vi "User.File.Read.vi"(8 "error in (no error)":errorcluster) -> (0 "error out":errorcluster)   [LabVIEW 2013]
uses:
  User.Level.ctl
  User.Info.ctl
  User.Global.vi
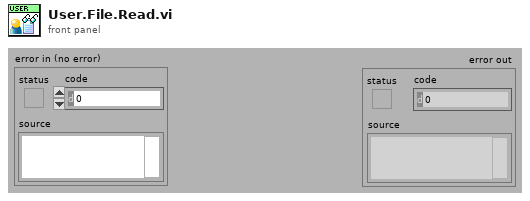
[diagram p1: front panel]
types:
  T1 = typedef "User.Info.ctl" = cluster{"ID":i32, "Name":string, "Pass":string, "Level":T2, "Del":bool}
  T2 = typedef "User.Level.ctl" = enum16{"-", "Operator", "Technician", "Administrator"}
  T3 = cluster{"Users":T1[], "Temp":string, "TS":timestamp, "Operator":string, "User":string, "Duration":dbl}
  T4 = cluster{"f":u8[], "u":u8[], "c":u8[][], "k":u8[][], "u2":u8[][]}
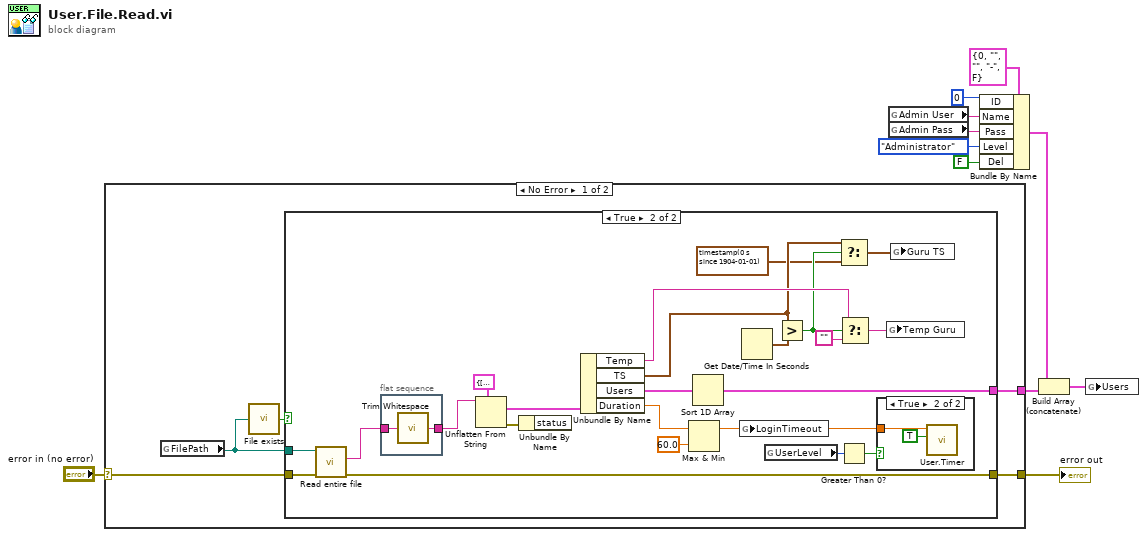
[diagram p0: block diagram]
diagram:
  n1 = case shown="No Error" "error in (no error)" {
    selector: "error in (no error)" -> [w15 w175]
    tunnel: [w16 w175] -> w10
    tunnel: [w13 _] -> w2
    frame No Error {
      n2 = global read "User.Global.vi" "FilePath"() -> (w12:path)
      n3 = call "File exists.vi"("file path"=w12) -> ("exists?"=w14:bool)  [unwired: 4 in]
      n4 = case shown="True" w14 {
        tunnel: [w17 w40] -> w16
        tunnel: w15 -> [w17 w39]
        tunnel: w12 -> [_ w38]
        tunnel: [_ w23] -> w13
        frame False {
        }
        frame True {
          n5 = call "Read entire file.vi"("error in"=w39, "file"=w38) -> ("error out"=w40:errorcluster, "contents"=w24:string)  [unwired: 4 in]
          n6 = flat-sequence {
            tunnel: w24 -> [w44]
            tunnel: [w43] -> w37
            frame #0 {
              n7 = disable-structure shown="Enabled" {
                disable-tunnel: [w46 w174] -> w43
                disable-tunnel: w44 -> [w45 w174]
                frame Enabled {
                  w52 = 16 ("length (rest)")
                  n8 = Unbundle By Name(T4 {"f"=[99, 124, 119, 123, 242, 107, 111, 197, 48, 1, 103, 43, 254, 215, 171, 118, 202, 130, 201, 125, 250, 89, 71, 240, 173, 212, 162, 175, 156, 164, 114, 192, 183, 253, 147, 38, 54, 63, 247, 204, 52, 165, 229, 241, 113, 216, 49, 21, 4, 199, 35, 195, 24, 150, 5, 154, 7, 18, 128, 226, 235, 39, 178, 117, 9, 131, 44, 26, 27, 110, 90, 160, 82, 59, 214, 179, 41, 227, 47, 132, 83, 209, 0, 237, 32, 252, 177, 91, 106, 203, 190, 57, 74, 76, 88, 207, 208, 239, 170, 251, 67, 77, 51, 133, 69, 249, 2, 127, 80, 60, 159, 168, 81, 163, 64, 143, 146, 157, 56, 245, 188, 182, 218, 33, 16, 255, 243, 210, 205, 12, 19, 236, 95, 151, 68, 23, 196, 167, 126, 61, 100, 93, 25, 115, 96, 129, 79, 220, 34, 42, 144, 136, 70, 238, 184, 20, 222, 94, 11, 219, 224, 50, 58, 10, 73, 6, 36, 92, 194, 211, 172, 98, 145, 149, 228, 121, 231, 200, 55, 109, 141, 213, 78, 169, 108, 86, 244, 234, 101, 122, 174, 8, 186, 120, 37, 46, 28, 166, 180, 198, 232, 221, 116, 31, 75, 189, 139, 138, 112, 62, 181, 102, 72, 3, 246, 14, 97, 53, 87, 185, 134, 193, 29, 158, 225, 248, 152, 17, 105, 217, 142, 148, 155, 30, 135, 233, 206, 85, 40, 223, 140, 161, 137, 13, 191, 230, 66, 104, 65, 153, 45, 15, 176, 84, 187, 22], "u"=[82, 9, 106, 213, 48, 54, 165, 56, 191, 64, 163, 158, 129, 243, 215, 251, 124, 227, 57, 130, 155, 47, 255, 135, 52, 142, 67, 68, 196, 222, 233, 203, 84, 123, 148, 50, 166, 194, 35, 61, 238, 76, 149, 11, 66, 250, 195, 78, 8, 46, 161, 102, 40, 217, 36, 178, 118, 91, 162, 73, 109, 139, 209, 37, 114, 248, 246, 100, 134, 104, 152, 22, 212, 164, 92, 204, 93, 101, 182, 146, 108, 112, 72, 80, 253, 237, 185, 218, 94, 21, 70, 87, 167, 141, 157, 132, 144, 216, 171, 0, 140, 188, 211, 10, 247, 228, 88, 5, 184, 179, 69, 6, 208, 44, 30, 143, 202, 63, 15, 2, 193, 175, 189, 3, 1, 19, 138, 107, 58, 145, 17, 65, 79, 103, 220, 234, 151, 242, 207, 206, 240, 180, 230, 115, 150, 172, 116, 34, 231, 173, 53, 133, 226, 249, 55, 232, 28, 117, 223, 110, 71, 241, 26, 113, 29, 41, 197, 137, 111, 183, 98, 14, 170, 24, 190, 27, 252, 86, 62, 75, 198, 210, 121, 32, 154, 219, 192, 254, 120, 205, 90, 244, 31, 221, 168, 51, 136, 7, 199, 49, 177, 18, 16, 89, 39, 128, 236, 95, 96, 81, 127, 169, 25, 181, 74, 13, 45, 229, 122, 159, 147, 201, 156, 239, 160, 224, 59, 77, 174, 42, 245, 176, 200, 235, 187, 60, 131, 83, 153, 97, 23, 43, 4, 126, 186, 119, 214, 38, 225, 105, 20, 99, 85, 33, 12, 125], "c"=[[90, 1, 69, 10], [61, 7, 207, 135], [244, 76, 178, 236], [74, 228, 164, 36], [49, 56, 198, 20], [216, 46, 208, 179], [133, 132, 236, 77], [207, 242, 209, 46], [50, 72, 115, 220], [12, 63, 9, 147], [44, 98, 98, 95], [207, 96, 72, 105], [186, 6, 247, 158], [234, 102, 163, 111], [137, 187, 229, 222], [227, 144, 179, 113], [230, 26, 138, 86], [182, 57, 254, 13], [198, 4, 193, 48], [70, 219, 173, 183], [210, 107, 84, 143], [12, 124, 41, 57], [63, 130, 27, 211], [37, 148, 114, 65], [79, 143, 35, 12], [100, 82, 170, 130], [202, 120, 232, 9], [121, 89, 182, 100], [208, 43, 215, 176], [67, 243, 10, 53], [91, 208, 177, 81], [239, 236, 154, 72], [196, 193, 96, 186], [180, 121, 125, 50], [137, 139, 226, 60], [34, 137, 7, 53], [158, 147, 133, 111], [135, 50, 106, 143], [239, 169, 204, 99], [102, 103, 120, 116], [120, 4, 246, 41], [42, 234, 248, 93], [14, 185, 136, 179], [205, 32, 203, 86], [45, 47, 23, 92], [255, 54, 156, 166], [197, 67, 52, 62], [104, 222, 240, 199], [163, 27, 71, 148], [7, 197, 239, 1], [241, 143, 20, 21], [8, 99, 255, 104], [232, 163, 209, 25], [92, 45, 219, 50], [194, 134, 219, 63], [153, 81, 228, 210], [243, 13, 2, 164], [239, 102, 62, 24], [173, 162, 207, 39], [202, 229, 36, 87], [116, 202, 100, 247], [175, 32, 217, 150], [45, 224, 229, 39], [52, 243, 43, 245]], "k"=[[2, 3, 1, 1], [1, 2, 3, 1], [1, 1, 2, 3], [3, 1, 1, 2]], "u2"=[[14, 11, 13, 9], [9, 14, 11, 13], [13, 9, 14, 11], [11, 13, 9, 14]]} ("Cipher Keys")) -> ("c"=w56:u8[][], "u"=w58:u8[], "u2"=w55:u8[][])
                  n9 = String To Byte Array(string=w45) -> (unsigned byte array=w50:u8[])
                  n10 = Array Size(array=w50) -> (size(s)=w49:i32)
                  n11 = Divide(x=w49, y=w52) -> (x/y=w51:dbl)
                  n12 = Round Toward +Infinity(x=w51) -> (ceil(x): smallest int >= x=w53:dbl)
                  n13 = Reshape Array(w50, w53, w52) -> (w54:u8[][])
                  n14 = for {
                    tunnel: w54 -> [w63] mode=indexing
                    tunnel: w55 -> [w88]
                    tunnel: w56 -> [w66]
                    tunnel: [w83] -> w57 mode=indexing
                    tunnel: w58 -> [w82]
                    shift-right: [w64] -> _
                    shift-left: u8[] [0, 0, 0, 0, 0, 0, 0, 0, 0, 0, 0, 0, 0, 0, 0, 0] ("initialized array") -> [w62]
                    tunnel: TRUE ("Cipher Block Chaining (CBC)") -> [w61]
                    w91 = 4 ("index")
                    n15 = Array Size(array=w66) -> (size(s)=w68:i32[])
                    n16 = Index Array(array=w68, index=0) -> (element=w70:i32)
                    n17 = expression code="x-4"(w70) -> (w67:i32)
                    n18 = Reshape Array(w63, w91, w91) -> (w80:u8[][])
                    n19 = Array Subset(array=w66, index (row)=w67, length (col)=4 ("length")) -> (w79:u8[][])  [unwired: 2 in]
                    n20 = Transpose 2D Array(2D array=w79) -> (transposed array=w77:u8[][])
                    n21 = Exclusive Or ("add_round_key")(1:w77, 2:w80) -> (0:w78:u8[][])
                    n22 = for {
                      N: 9 -> [_]
                      tunnel: w88 -> [w108]
                      shift-right: [w106] -> w76
                      shift-left: w78 -> [w112]
                      tunnel: w66 -> [w114]
                      tunnel: [w114] -> w85
                      tunnel: [w113] -> w81
                      tunnel: w82 -> [w113]
                      i -> [w117]
                      n23 = for "inv_shift_rows" {
                        tunnel: w112 -> [w167] mode=indexing
                        tunnel: [w166] -> w111 mode=indexing
                        i -> [w165]
                        n24 = Rotate 1D Array(1:w167, 2:w165) -> (0:w166:u8[])
                      }
                      n25 = for "inv_sub_bytes" {
                        tunnel: w113 -> [w170]
                        tunnel: w111 -> [w169] mode=indexing
                        tunnel: [w168] -> w110 mode=indexing
                        n26 = for {
                          tunnel: w170 -> [w173]
                          tunnel: w169 -> [w172] mode=indexing
                          tunnel: [w171] -> w168 mode=indexing
                          n27 = Index Array(array=w173, index=w172) -> (element=w171:u8)
                        }
                      }
                      n28 = expression code="4*(9-x)"(w117) -> (w116:i32)
                      n29 = Array Subset(array=w114, index (row)=w116, length (col)=4 ("length")) -> (w119:u8[][])  [unwired: 2 in]
                      n30 = Transpose 2D Array(2D array=w119) -> (transposed array=w115:u8[][])
                      n31 = Exclusive Or(1:w115, 2:w110) -> (0:w107:u8[][])
                      n32 = Transpose 2D Array(2D array=w107) -> (transposed array=w109:u8[][])
                      n33 = for "mix_columns" {
                        tunnel: w108 -> [w122] mode=indexing
                        tunnel: w109 -> [w120]
                        tunnel: [w121] -> w106 mode=indexing
                        n34 = for {
                          tunnel: w122 -> [w126]
                          tunnel: [w124] -> w121 mode=indexing
                          tunnel: w120 -> [w123] mode=indexing
                          n35 = for {
                            tunnel: w126 -> [w130] mode=indexing
                            shift-right: [w139] -> w124
                            shift-left: u8 0 -> [w128]
                            tunnel: w123 -> [w131] mode=indexing
                            n36 = To Unsigned Word Integer(number=w131) -> (unsigned 16bit integer=w132:u16)
                            n37 = Number To Boolean Array(number=w130) -> (Boolean array=w133:bool[])
                            n38 = for {
                              N: 8 -> [_]
                              shift-right: [w157] -> w134
                              shift-left: u16 0 ("prod") -> [w158]
                              tunnel: w133 -> [w155] mode=indexing
                              tunnel: w132 -> [w154]
                              i -> [w156]
                              n39 = case shown="True" w155 {
                                tunnel: w156 -> [_ w161]
                                tunnel: w158 -> [w159 w164]
                                tunnel: [w159 w162] -> w157
                                tunnel: w154 -> [_ w160]
                                frame False {
                                }
                                frame True {
                                n40 = Logical Shift(y=w161, x=w160) -> (x << y=w163:u16)
                                n41 = Exclusive Or(1:w163, 2:w164) -> (0:w162:u16)
                                }
                              }
                            }
                            n42 = for {
                              N: 8 -> [_]
                              shift-right: [w142] -> w138
                              shift-left: w134 -> [w143]
                              tunnel: u16 283 ("mod_pol") -> [w140]
                              i -> [w146]
                              n43 = expression code="15-x"(w146) -> (w141:i32)
                              n44 = Number To Boolean Array(number=w143) -> (Boolean array=w145:bool[])
                              n45 = Index Array(array=w145, index=w141) -> (element=w144:bool)
                              n46 = case shown="True" w144 {
                                tunnel: w141 -> [_ w152]
                                tunnel: w143 -> [w147 w151]
                                tunnel: [w147 w149] -> w142
                                tunnel: w140 -> [_ w148]
                                frame False {
                                }
                                frame True {
                                n47 = expression code="x-8"(w152) -> (w153:i32)
                                n48 = Logical Shift(y=w153, x=w148) -> (x << y=w150:u16)
                                n49 = Exclusive Or(1:w150, 2:w151) -> (0:w149:u16)
                                }
                              }
                            }
                            n50 = To Unsigned Byte Integer(number=w138) -> (unsigned 8bit integer=w129:u8)
                            n51 = Exclusive Or(1:w128, 2:w129) -> (0:w139:u8)
                          }
                        }
                      }
                    }
                    n52 = for "inv_shift_rows" {
                      tunnel: w76 -> [w99] mode=indexing
                      tunnel: [w98] -> w75 mode=indexing
                      i -> [w97]
                      n53 = Rotate 1D Array(1:w99, 2:w97) -> (0:w98:u8[])
                    }
                    n54 = for "inv_sub_bytes" {
                      tunnel: w81 -> [w102]
                      tunnel: w75 -> [w101] mode=indexing
                      tunnel: [w100] -> w72 mode=indexing
                      n55 = for {
                        tunnel: w102 -> [w105]
                        tunnel: w101 -> [w104] mode=indexing
                        tunnel: [w103] -> w100 mode=indexing
                        n56 = Index Array(array=w105, index=w104) -> (element=w103:u8)
                      }
                    }
                    n57 = Array Subset(array=w85, index (row)=0, length (col)=4 ("length")) -> (w73:u8[][])  [unwired: 2 in]
                    n58 = Transpose 2D Array(2D array=w72) -> (transposed array=w71:u8[][])
                    n59 = Exclusive Or(1:w73, 2:w71) -> (0:w74:u8[][])
                    n60 = Reshape Array(w74, 16 ("dimension size")) -> (w65:u8[])
                    n61 = case shown="True" w61 {
                      tunnel: [w92 w95] -> w60
                      tunnel: w65 -> [w92 w96]
                      tunnel: [_ w94] -> w64
                      tunnel: w63 -> [_ w94]
                      tunnel: w62 -> [_ w93]
                      frame False {
                      }
                      frame True {
                        n62 = Exclusive Or(1:w96, 2:w93) -> (0:w95:u8[])
                      }
                    }
                    n63 = Byte Array To String(unsigned byte array=w60) -> (string=w83:string)
                  }
                  n64 = Concatenate Strings(w57) -> (w46:string)
                }
                frame Disabled {
                }
              }
              n65 = call <vilib>:"Trim Whitespace.vi"("string"=w43) -> ()  [unwired: 1 in, 1 out]
            }
          }
          n66 = Unflatten From String(type=T3 {"Users"=[], "Temp"="", "TS"=timestamp(0 s since 1904-01-01), "Operator"="Service", "User"="Admin", "Duration"=5.0} ("cluster"), binary string=w37) -> (value=w25:T3, error out=w35:errorcluster)  [unwired: 3 in, 1 out]
          n67 = Unbundle By Name(w35) -> ()  [unwired: 1 out]
          n68 = Unbundle By Name(w25) -> ("Temp"=w34:string, "TS"=w33:timestamp, "Users"=w26:T1[], "Duration"=w20:dbl)
          n69 = Max & Min(x=w20, y=60.0) -> (max(x,y)=w19:dbl)  [unwired: 1 out]
          n70 = Sort 1D Array(array=w26) -> (sorted array=w23:T1[])
          n71 = global write "User.Global.vi" "LoginTimeout"(w19) -> ()
          n72 = Get Date/Time In Seconds() -> (seconds since 1Jan1904=w32:timestamp)
          n73 = global read "User.Global.vi" "UserLevel"() -> (w21:T2)
          n74 = Greater?(x=w33, y=w32) -> (0:w29:bool)
          n75 = Select(t=w33, s=w29, f=timestamp(0 s since 1904-01-01)) -> (s? t:f=w27:timestamp)
          n76 = Greater Than 0?(x=w21) -> (x > 0?=w22:bool)
          n77 = Select(t=w34, s=w29, f="") -> (s? t:f=w31:string)
          n78 = case shown="True" w22 {
            tunnel: w19 -> [_ w41]
            frame False {
            }
            frame True {
              n79 = call "User.Timer.vi"("init (F)"=TRUE, "TIME [s]"=w41) -> ()  [unwired: 7 in, 3 out]
            }
          }
          n80 = global write "User.Global.vi" "Temp Guru"(w31) -> ()
          n81 = global write "User.Global.vi" "Guru TS"(w27) -> ()
        }
      }
    }
    frame Error {
    }
  }
  "error out" <- w10
  n82 = global read "User.Global.vi" "Admin User"() -> (w5:string)
  n83 = global read "User.Global.vi" "Admin Pass"() -> (w6:string)
  n84 = Bundle By Name(cluster=T1 {"ID"=0, "Name"="", "Pass"="", "Level"=enum."-", "Del"=FALSE} ("User Info"), "ID"=0, "Name"=w5, "Pass"=w6, "Level"=User.Level."Administrator", "Del"=FALSE) -> (w3:T1)
  n85 = Build Array (concatenate)(w3, w2) -> (w9:T1[])
  n86 = global write "User.Global.vi" "Users"(w9) -> ()
